vi "Run Inject.vi"(7 "auto_switch_valve":bool=TRUE, 8 "error in (no error)":errorcluster, 11 "PHD Ultra in":refnum<class "PHD Ultra.lvclass">) -> (0 "error out":errorcluster, 3 "PHD Ultra out":refnum<class "PHD Ultra.lvclass">)   [LabVIEW 2018, in "PHD Ultra.lvlib" / "PHD Ultra.lvclass"]
uses:
  PHD Ultra.lvclass
  Resources/GLOBAL/GLOBAL Time-critical.vi
  <userlib>/QmixLib/QmixLib.lvlib
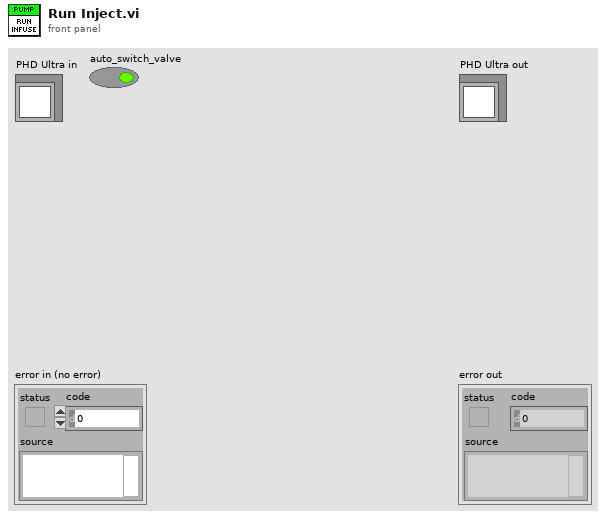
[diagram p1: front panel]
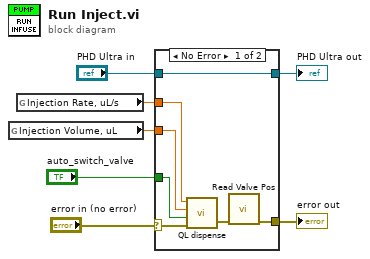
[diagram p0: block diagram]
diagram:
  n1 = global read "GLOBAL Time-critical.vi" "Injection Volume, uL"() -> (w2:dbl)
  n2 = global read "GLOBAL Time-critical.vi" "Injection Rate, uL/s"() -> (w1:dbl)
  n3 = case shown="No Error" "error in (no error)" {
    selector: "error in (no error)" -> [w13 w16]
    tunnel: [w8 w16] -> w6
    tunnel: [w14 w15] -> w4
    tunnel: "PHD Ultra in" -> [w14 w15]
    tunnel: w2 -> [w12 _]
    tunnel: "auto_switch_valve" -> [w11 _]
    tunnel: w1 -> [w10 _]
    frame No Error {
      n4 = call <userlib>:"QL dispense.vi"("error in (no error)"=w13, "auto_switch_valve"=w11, "volume_uL"=w12, "flow_rate_uL_s"=w10) -> ("error out"=w9:errorcluster)  [unwired: 3 in]
      n5 = call "Read Valve Pos.vi"("error in (no error)"=w9) -> ("error out"=w8:errorcluster)  [unwired: 10 in]
    }
    frame Error {
    }
  }
  "error out" <- w6
  "PHD Ultra out" <- w4
